vi "DSF.Engine.Plugin.Create.vi"(5 "Debug Flags":refnum<class "Debug Flags.lvclass">, 7 "transceiver count":i32, 8 "error in (no error)":errorcluster, 9 "component classes":refnum<class>[](array[class]), 10 "Plugin Configuration":refnum<class "Plugin Configuration.lvclass">, 11 "Transfer Groups":refnum<class "DSF.Engine.Transfer Group.lvclass">[](array[class])) -> (0 "error out":errorcluster, 2 "Transceiver":refnum<class "DSF.Engine.Transceiver.lvclass">, 3 "Plugin out":refnum<class "DSF.Engine.Plugin.lvclass">)   [LabVIEW 2017, in "Data Sharing Framework Engine.lvlib" / "DSF.Engine.Plugin.lvclass"]
uses:
  DSF.Engine.Plugin.lvclass
  Transfer/DSF.Engine.Transfer Group.lvclass
  Source/Data Sharing Framework Core/Engine/Debug/Debug Flags/Debug Flags.lvclass
  Source/Data Sharing Framework Core/Engine/Configuration Classes/Plugin Configuration/Plugin Configuration.lvclass
  C:/github/data-sharing-framework/Source/Data Sharing Framework Core/Engine/Configuration Classes/Configuration/Configuration.lvclass
  Transceiver/DSF.Engine.Transceiver.lvclass
  Source/Data Sharing Framework Core/Engine/Configuration Classes/Configuration/Configuration.lvclass/Configuration.ctl
  Source/Data Sharing Framework Core/Engine/Configuration Classes/Plugin Configuration/Plugin Configuration.lvclass/Plugin Configuration.ctl
  DSF.Engine.Plugin.lvclass/DSF.Engine.Plugin.ctl
  Timing/DSF.Engine.Timing.lvclass
  Source/Data Sharing Framework Core/Engine/Configuration Classes/Configuration/Configuration.lvclass
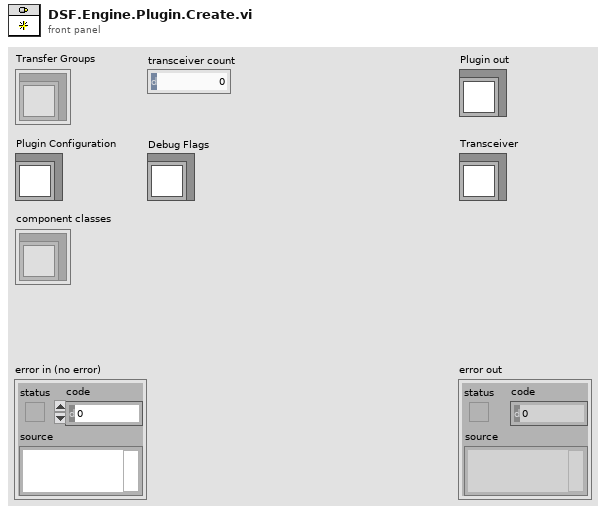
[diagram p1: front panel]
types:
  T1 = typedef "DSF Configuration API.lvlib/DSF Timing Info.ctl" = cluster{"priority":u64, "decimation":u64, "offset":u64}
  T2 = typedef "DSF Configuration API.lvlib/DSF Settings Info.ctl" = cluster{"key":string, "value":string}[]
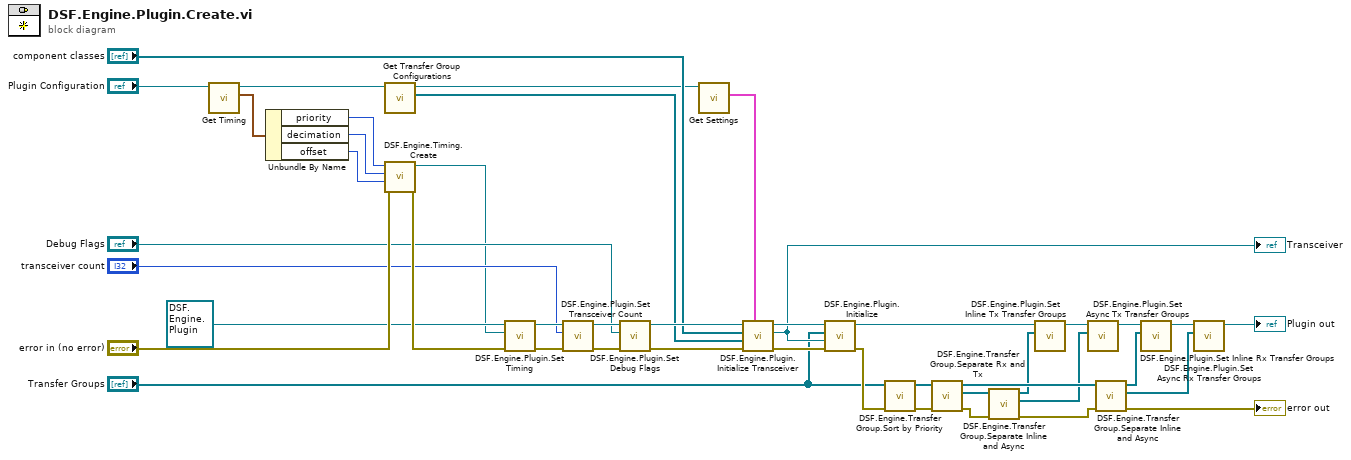
[diagram p0: block diagram]
diagram:
  n1 = call "Get Timing.vi"("Plugin Configuration in"="Plugin Configuration") -> ("cycle timing"=w16:T1, "Plugin Configuration out"=w11:refnum<class "Plugin Configuration.lvclass">)  [unwired: 9 in]
  n2 = Unbundle By Name(w16) -> ("priority"=w13:u64, "decimation"=w14:u64, "offset"=w15:u64)
  n3 = call "Get Transfer Group Configurations.vi"("Plugin Configuration in"=w11) -> ("Transfer Group Configurations"=w6:refnum<class "Transfer Group Configuration.lvclass">[], "Plugin Configuration out"=w2:refnum<class "Plugin Configuration.lvclass">)  [unwired: 9 in]
  n4 = call "DSF.Engine.Timing.Create.vi"("error in (no error)"="error in (no error)", "Offset"=w15, "Decimation"=w14, "Priority"=w13) -> ("error out"=w39:errorcluster, "Timing"=w10:refnum<class "DSF.Engine.Timing.lvclass">)  [unwired: 6 in]
  n5 = call "DSF.Engine.Plugin.Set Timing.vi"("Timing"=w10, "Plugin in"=refnum<class "DSF.Engine.Plugin.lvclass"> refnum) -> ("Plugin out"=w36:refnum<class "DSF.Engine.Plugin.lvclass">)  [unwired: 9 in]
  n6 = call "DSF.Engine.Plugin.Set Transceiver Count.vi"("transceiver count"="transceiver count", "Plugin in"=w36) -> ("Plugin out"=w23:refnum<class "DSF.Engine.Plugin.lvclass">)  [unwired: 9 in]
  n7 = call "DSF.Engine.Plugin.Set Debug Flags.vi"("Debug Flags"="Debug Flags", "Plugin in"=w23) -> ("Plugin out"=w9:refnum<class "DSF.Engine.Plugin.lvclass">)  [unwired: 9 in]
  n8 = call "Get Settings.vi"("Configuration in"=w2) -> ("settings"=w1:T2)  [unwired: 9 in, 1 out]
  n9 = call "DSF.Engine.Plugin.Initialize Transceiver.vi"("transceiver settings"=w1, "error in (no error)"=w39, "Transfer Groups Configurations"=w6, "component classes"="component classes", "Plugin in"=w9) -> ("error out"=w4:errorcluster, "Transceiver"=w5:refnum<class "DSF.Engine.Transceiver.lvclass">, "Plugin out"=w8:refnum<class "DSF.Engine.Plugin.lvclass">)  [unwired: 4 in]
  "Transceiver" <- w5
  n10 = call "DSF.Engine.Plugin.Initialize.vi"("error in (no error)"=w4, "Transceiver"=w5, "Transfer Groups"="Transfer Groups", "Plugin in"=w8) -> ("error out"=w19:errorcluster, "Plugin out"=w21:refnum<class "DSF.Engine.Plugin.lvclass">)  [unwired: 6 in]
  n11 = call "DSF.Engine.Transfer Group.Sort by Priority.vi"("error in (no error)"=w19, "Transfer Groups"="Transfer Groups") -> ("error out"=w38:errorcluster, "sorted Transfer Groups"=w37:refnum<class "DSF.Engine.Transfer Group.lvclass">[])  [unwired: 8 in]
  n12 = call "DSF.Engine.Transfer Group.Separate Rx and Tx.vi"("error in (no error)"=w38, "Transfer Groups"=w37) -> ("error out"=w34:errorcluster, "Tx Transfer Groups"=w33:refnum<class "DSF.Engine.Transfer Group.lvclass">[], "Rx Transfer Groups"=w32:refnum<class "DSF.Engine.Transfer Group.lvclass">[])  [unwired: 7 in]
  n13 = call "DSF.Engine.Transfer Group.Separate Inline and Async.vi"("error in (no error)"=w34, "Transfer Groups"=w33) -> ("error out"=w31:errorcluster, "Async Transfer Groups"=w29:refnum<class "DSF.Engine.Transfer Group.lvclass">[], "Inline Transfer Groups"=w30:refnum<class "DSF.Engine.Transfer Group.lvclass">[])  [unwired: 7 in]
  n14 = call "DSF.Engine.Plugin.Set Inline Tx Transfer Groups.vi"("Inline Tx Transfer Groups"=w30, "Plugin in"=w21) -> ("Plugin out"=w28:refnum<class "DSF.Engine.Plugin.lvclass">)  [unwired: 9 in]
  n15 = call "DSF.Engine.Plugin.Set Async Tx Transfer Groups.vi"("Async Tx Transfer Groups"=w29, "Plugin in"=w28) -> ("Plugin out"=w26:refnum<class "DSF.Engine.Plugin.lvclass">)  [unwired: 9 in]
  n16 = call "DSF.Engine.Transfer Group.Separate Inline and Async.vi"("error in (no error)"=w31, "Transfer Groups"=w32) -> ("error out"=→"error out":errorcluster, "Async Transfer Groups"=w24:refnum<class "DSF.Engine.Transfer Group.lvclass">[], "Inline Transfer Groups"=w27:refnum<class "DSF.Engine.Transfer Group.lvclass">[])  [unwired: 7 in]
  n17 = call "DSF.Engine.Plugin.Set Inline Rx Transfer Groups.vi"("Inline Rx Transfer Groups"=w27, "Plugin in"=w26) -> ("Plugin out"=w25:refnum<class "DSF.Engine.Plugin.lvclass">)  [unwired: 9 in]
  n18 = call "DSF.Engine.Plugin.Set Async Rx Transfer Groups.vi"("Async Rx Transfer Groups"=w24, "Plugin in"=w25) -> ("Plugin out"=→"Plugin out":refnum<class "DSF.Engine.Plugin.lvclass">)  [unwired: 9 in]
